vi "ProcessTest_Data.vi"() -> (3 "Array":sgl[][](array[numeric]))   [LabVIEW 2020]
panel:
  out "x .and. y?":bool
  out "array":dbl[](array[numeric])
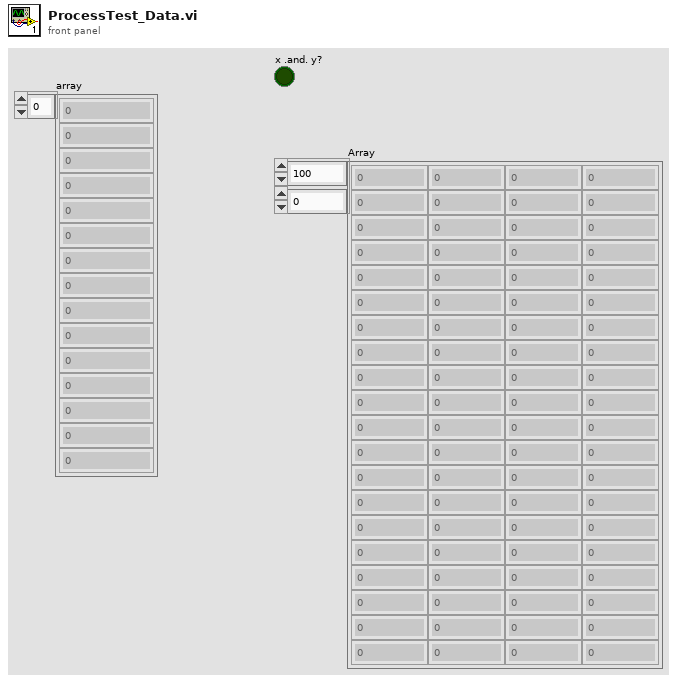
[diagram p1: front panel]
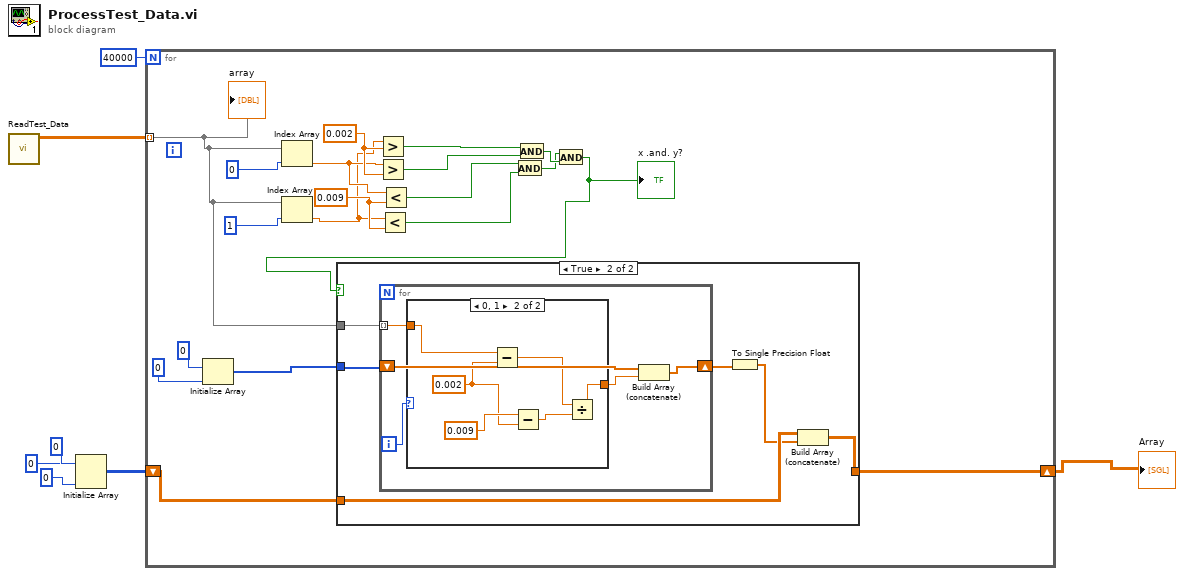
[diagram p0: block diagram]
diagram:
  n1 = call "ReadTest_Data.vi"() -> ("array"=w1:dbl[][])  [unwired: 11 in]
  n2 = Initialize Array(0, 0, 0) -> (w4:i32[][])
  n3 = for {
    N: 40000 -> [_]
    tunnel: w1 -> [w19] mode=indexing
    shift-right: [w17] -> w3
    shift-left: w4 -> [w18]
    w23 = 0.002
    w24 = 0.009
    n4 = Initialize Array(0, 0) -> (w20:i32[])
    n5 = Index Array(array=w19, index=0) -> (element=w9:dbl)
    n6 = Index Array(array=w19, index=1) -> (element=w8:dbl)
    n7 = Greater?(x=w8, y=w23) -> (0:w16:bool)
    n8 = Greater?(x=w9, y=w23) -> (0:w15:bool)
    n9 = Less?(x=w8, y=w24) -> (x < y?=w13:bool)
    n10 = Less?(x=w9, y=w24) -> (x < y?=w14:bool)
    n11 = And(x=w14, y=w13) -> (x .and. y?=w11:bool)
    n12 = And(x=w16, y=w15) -> (x .and. y?=w12:bool)
    n13 = And(x=w11, y=w12) -> (x .and. y?=w10:bool)
    "x .and. y?" <- w10
    n14 = case shown="True" w10 {
      tunnel: w20 -> [_ w32]
      tunnel: w19 -> [_ w33]
      tunnel: w18 -> [w27 w30]
      tunnel: [w27 w28] -> w17
      frame False {
      }
      frame True {
        n15 = for {
          tunnel: w33 -> [w37] mode=indexing
          shift-right: [w36] -> w31
          shift-left: w32 -> [w38]
          i -> [w34]
          n16 = case shown="0, 1" w34 {
            tunnel: w37 -> [w39 w41]
            tunnel: [w39 w40] -> w35
            frame Default {
            }
            frame 0, 1 {
              w43 = 0.002
              n17 = Subtract(x=w41, y=w43) -> (x-y=w45:dbl)
              n18 = Subtract(x=0.009, y=w43) -> (x-y=w42:dbl)
              n19 = Divide(x=w45, y=w42) -> (x/y=w40:dbl)
            }
          }
          n20 = Build Array (concatenate)(w38, w35) -> (w36:dbl[])
        }
        n21 = To Single Precision Float(number=w31) -> (single precision float=w29:sgl[])
        n22 = Build Array (concatenate)(w30, w29) -> (w28:sgl[][])
      }
    }
    "array" <- w19
  }
  "Array" <- w3
